vi "Get Name.vi"(8 "error in":errorcluster, 11 "Handler in":refnum<class "Handler.lvclass">) -> (0 "error out":errorcluster, 2 "Name":string, 3 "Handler out":refnum<class "Handler.lvclass">)   [LabVIEW 2016, in "hse-logger.lvlib" / "Handler.lvclass"]
doc: "Returns the ``Name`` of the Handler."
uses:
  Handler.lvclass
  Handler.lvclass/Handler.ctl
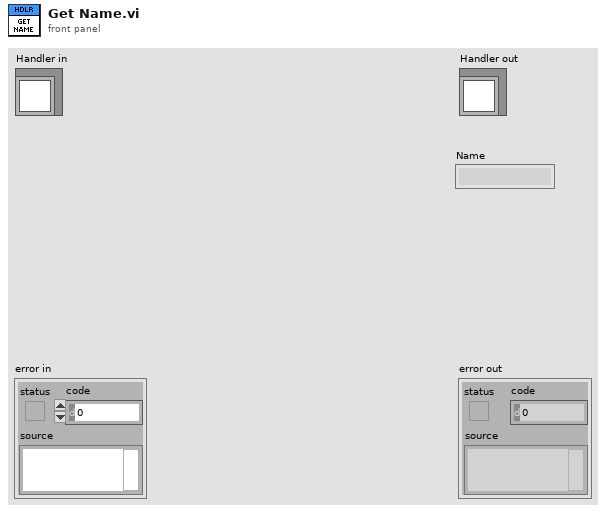
[diagram p1: front panel]
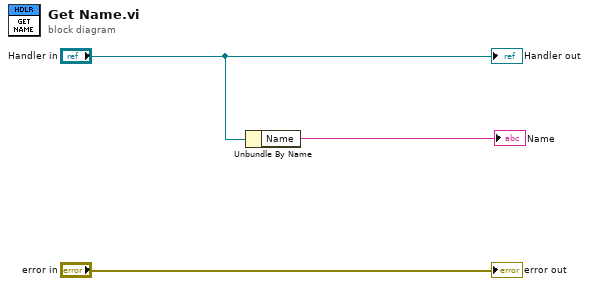
[diagram p0: block diagram]
diagram:
  n1 = Unbundle By Name("Handler in") -> ("Name"=→"Name":string)
  "error out" <- "error in"
  "Handler out" <- "Handler in"
